vi "RegisterArea.vi"(0 "Handle In":u64[](array[numeric]), 1 "error in (no error)":errorcluster, 5 "BitArea":u8[](array[numeric]), 7 "WordArea":u16[](array[numeric]), 9 "AreaID":T1(ring), 11 "Amount":i32) -> (3 "error out":errorcluster, 4 "Handle Out":u64[](array[numeric]), 6 "Result":i32)   [LabVIEW 2020, in "SnapMB.lvlib"]
uses:
  SnapMB.lvlib
  windows/snapmb.dll
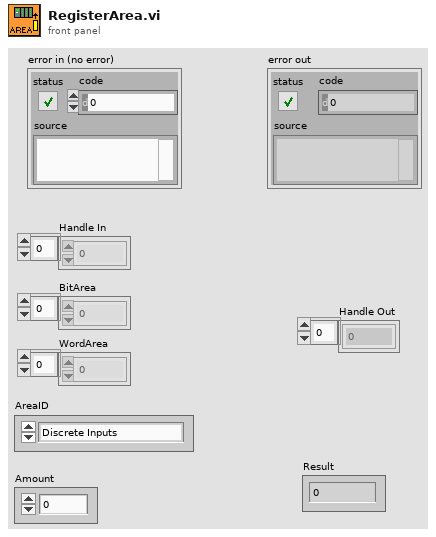
[diagram p1: front panel]
types:
  T1 = enum16{"Discrete Inputs", "Coils", "Input Registers", "Holding Registers"}
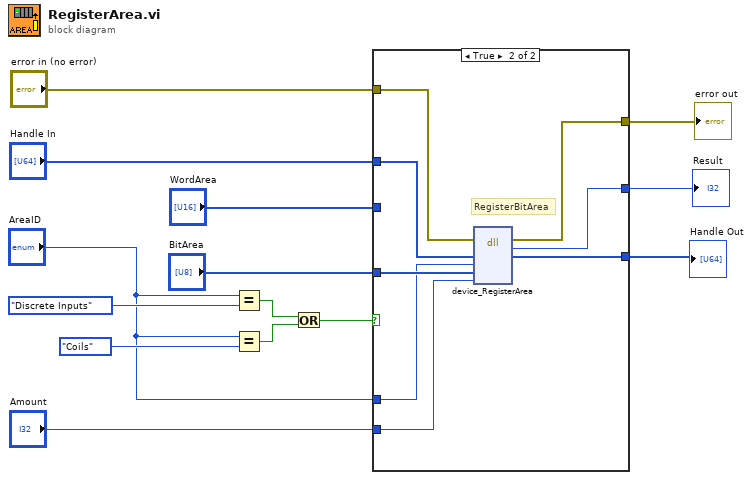
[diagram p0: block diagram]
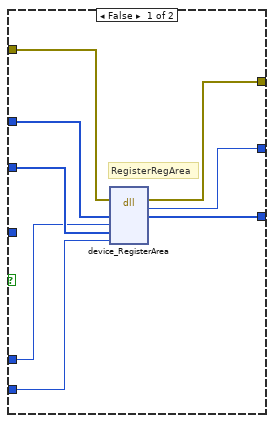
[diagram p2: hidden frame]
diagram:
  n1 = Equal?(x="AreaID", y=T1."Discrete Inputs") -> (x = y?=w12:bool)
  n2 = Equal?(x="AreaID", y=T1."Coils") -> (x = y?=w11:bool)
  n3 = Or(x=w12, y=w11) -> (x .or. y?=w10:bool)
  n4 = case shown="True" w10 {
    tunnel: "BitArea" -> [_ w30]
    tunnel: "WordArea" -> [w22 _]
    tunnel: "Handle In" -> [w21 w29]
    tunnel: "AreaID" -> [w20 w28]
    tunnel: "Amount" -> [w19 w27]
    tunnel: [w18 w26] -> w4
    tunnel: [w17 w25] -> w3
    tunnel: [w16 w24] -> w2
    tunnel: "error in (no error)" -> [w15 w23]
    frame False {
      # "RegisterRegArea"
      n5 = dll-call lib="D:/SnapMB/LabView/lib/windows/snapmb.dll" fn="device_RegisterArea"(error in=w15, "Device"=w21, "AreaID"=w20, "Data"=w22, "Amount"=w19) -> (error out=w16:errorcluster, "Result"=w17:i32, "Device"=w18:u64[])  [unwired: 5 in, 1 out]
    }
    frame True {
      # "RegisterBitArea"
      n6 = dll-call lib="D:/SnapMB/LabView/lib/windows/snapmb.dll" fn="device_RegisterArea"(error in=w23, "Device"=w29, "AreaID"=w28, "Data"=w30, "Amount"=w27) -> (error out=w24:errorcluster, "Result"=w25:i32, "Device"=w26:u64[])  [unwired: 5 in, 1 out]
    }
  }
  "Handle Out" <- w4
  "Result" <- w3
  "error out" <- w2
